vi "ma_MultitoneParamsCheck.vi"(4 "coerce frequencies?":bool, 5 "Relative error":dbl=1e-09 format="%0.3e", 6 "Phases":dbl[](array[numeric]) format="%0.2f", 7 "Samples":i32, 8 "error in (no error)":errorcluster, 9 "Sampling Rate":dbl format="%0.2f", 10 "Tone Frequencies":dbl[](array[numeric]) format="%0.2f", 11 "Tone Amplitudes":dbl[](array[numeric]) format="%0.2f") -> (0 "error out":errorcluster, 1 "Phases out":dbl[](array[numeric]) format="%0.2f", 2 "Tone Frequencies out":dbl[](array[numeric]) format="%0.2f", 3 "Tone Amplitudes out":dbl[](array[numeric]) format="%0.2f")   [LabVIEW 2020, in "NI_MAPro.lvlib"]
uses:
  NI_MAPro.lvlib
  NI_MABase.lvlib
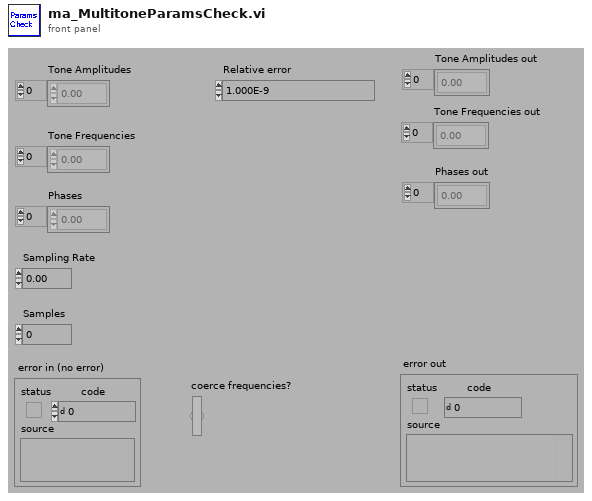
[diagram p1: front panel]
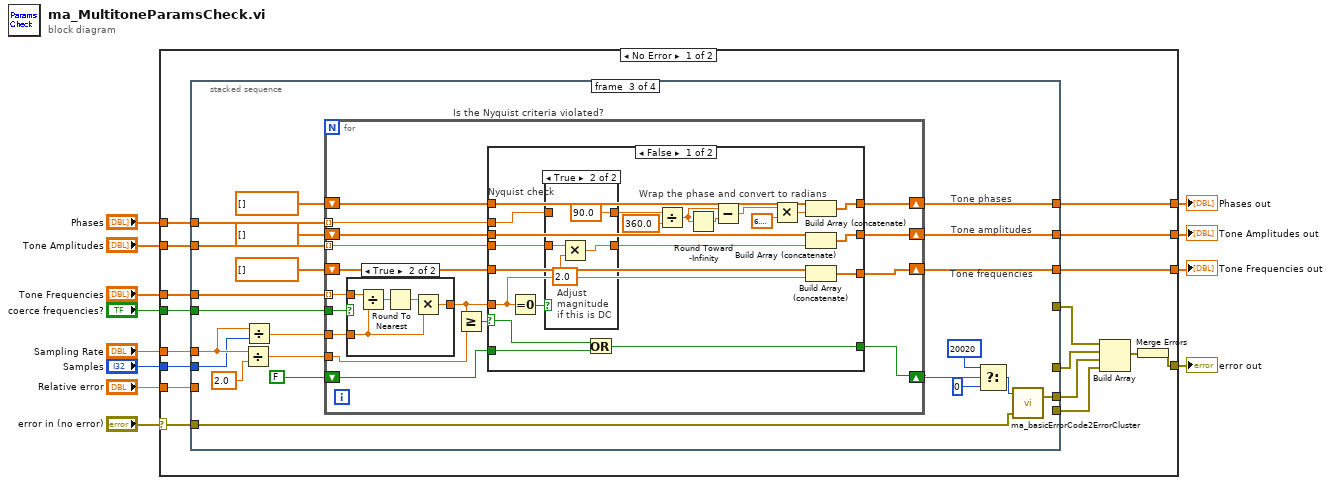
[diagram p0: block diagram]
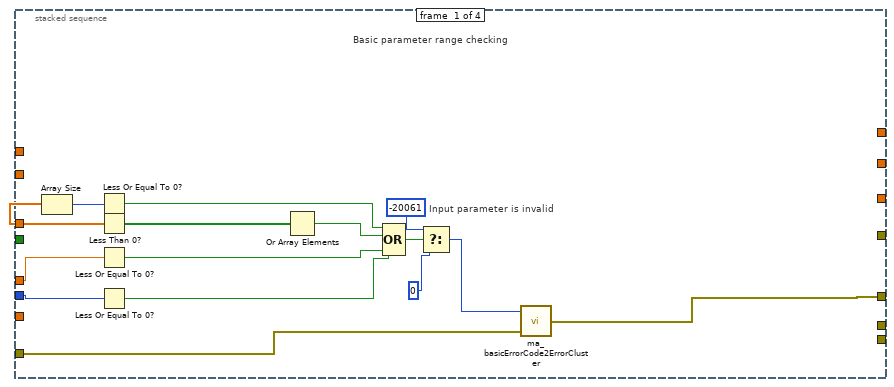
[diagram p2: hidden frame]
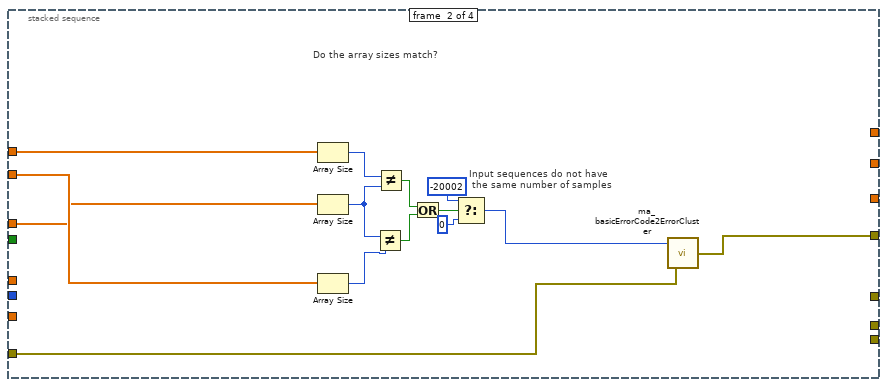
[diagram p3: hidden frame]
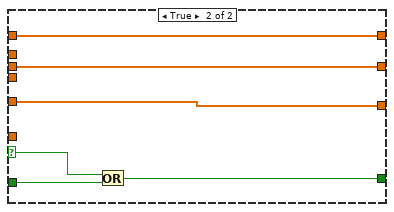
[diagram p6: hidden frame]
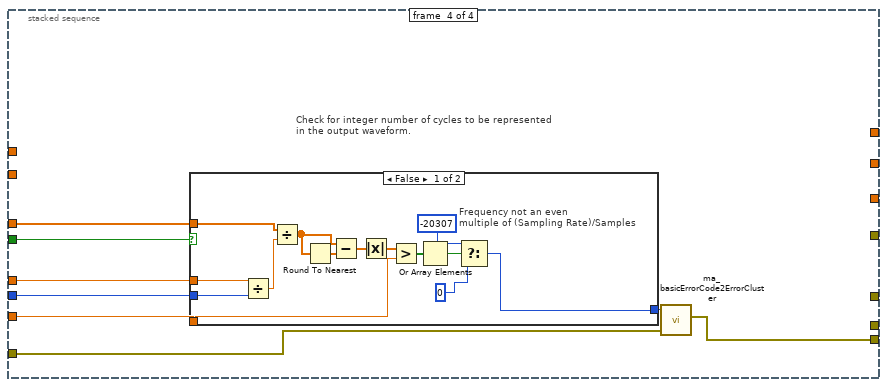
[diagram p7: hidden frame]
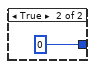
[diagram p8: hidden frame]
diagram:
  n1 = case shown="No Error" "error in (no error)" {
    selector: "error in (no error)" -> [w21 w159]
    tunnel: "Tone Frequencies" -> [w29 w160]
    tunnel: "Tone Amplitudes" -> [w28 w161]
    tunnel: "Sampling Rate" -> [w27 _]
    tunnel: "Samples" -> [w26 _]
    tunnel: "Phases" -> [w25 w162]
    tunnel: [w24 w162] -> w3
    tunnel: [w23 w161] -> w7
    tunnel: [w22 w160] -> w6
    tunnel: [w15 w159] -> w4
    tunnel: "Relative error" -> [w14 _]
    tunnel: "coerce frequencies?" -> [w13 _]
    frame No Error {
      n2 = stacked-sequence {
        tunnel: w29 -> [w34 w56 w80 w140]
        tunnel: w28 -> [_ w58 w79 _]
        tunnel: w27 -> [w43 _ w62 w143]
        tunnel: w26 -> [w44 _ w61 w142]
        tunnel: w14 -> [_ _ _ w141]
        tunnel: w25 -> [_ w57 w78 _]
        tunnel: [_ _ w67 _] -> w24
        tunnel: [_ _ w68 _] -> w23
        tunnel: [_ _ w71 _] -> w22
        tunnel: [w36 _ _ _] -> w19
        tunnel: w21 -> [w35 w50 w73 w139]
        tunnel: [_ w49 _ _] -> w20
        tunnel: [_ _ w72 _] -> w18
        tunnel: [_ _ _ w138] -> w17
        tunnel: w13 -> [_ _ w59 w136]
        frame #0 {
          # "Input parameter is invalid"
          # "Basic parameter range checking"
          n3 = Array Size(array=w34) -> (size(s)=w38:i32)
          n4 = Less Or Equal To 0?(x=w38) -> (x <= 0?=w37:bool)
          n5 = Less Than 0?(x=w34) -> (x < 0?=w42:bool[])
          n6 = Less Or Equal To 0?(x=w43) -> (x <= 0?=w41:bool)
          n7 = Less Or Equal To 0?(x=w44) -> (x <= 0?=w40:bool)
          n8 = Or Array Elements(Boolean array=w42) -> (logical OR=w39:bool)
          n9 = Compound Arithmetic op=OR(w37, w39, w41, w40) -> (w33:bool)
          n10 = Select(t=-20061 ("Bundle Element"), s=w33, f=0) -> (s? t:f=w30:i32)
          n11 = call "ma_basicErrorCode2ErrorCluster.vi"("error in (no error)"=w35, "Error Code"=w30) -> ("error out"=w36:errorcluster)  [unwired: 1 in]
        }
        frame #1 {
          # "Input sequences do not have\n the same number of samples"
          # "Do the array sizes match?"
          n12 = Array Size(array=w57) -> (size(s)=w52:i32)
          n13 = Array Size(array=w56) -> (size(s)=w53:i32)
          n14 = Array Size(array=w58) -> (size(s)=w51:i32)
          n15 = Not Equal?(x=w53, y=w51) -> (x != y?=w55:bool)
          n16 = Not Equal?(x=w52, y=w53) -> (x != y?=w54:bool)
          n17 = Or(x=w54, y=w55) -> (x .or. y?=w48:bool)
          n18 = Select(t=-20002 ("Bundle Element"), s=w48, f=0) -> (s? t:f=w45:i32)
          n19 = call "ma_basicErrorCode2ErrorCluster.vi"("error in (no error)"=w50, "Error Code"=w45) -> ("error out"=w49:errorcluster)  [unwired: 1 in]
        }
        frame #2 {
          # "Tone phases"
          # "Tone amplitudes"
          # "Tone frequencies"
          # "Is the Nyquist criteria violated?"
          # "Nyquist check"
          n20 = Divide(x=w62, y=2.0) -> (x/y=w69:dbl)
          n21 = Divide(x=w62, y=w61) -> (x/y=w60:dbl)
          n22 = for {
            tunnel: w69 -> [w85]
            tunnel: w80 -> [w84] mode=indexing
            shift-right: [w92] -> w71
            shift-left: dbl[] [] -> [w93]
            shift-right: [w94] -> w66
            shift-left: FALSE -> [w95]
            shift-right: [w89] -> w67
            shift-left: dbl[] [] -> [w90]
            shift-right: [w88] -> w68
            shift-left: dbl[] [] -> [w91]
            tunnel: w79 -> [w87] mode=indexing
            tunnel: w78 -> [w86] mode=indexing
            tunnel: w60 -> [w83]
            tunnel: w59 -> [w82]
            n23 = case shown="True" w82 {
              tunnel: w84 -> [w97 w102]
              tunnel: w83 -> [_ w99]
              tunnel: [w97 w98] -> w81
              frame False {
              }
              frame True {
                n24 = Divide(x=w102, y=w99) -> (x/y=w101:dbl)
                n25 = Round To Nearest(number=w101) -> (nearest integer value=w100:dbl)
                n26 = Multiply(x=w100, y=w99) -> (x*y=w98:dbl)
              }
            }
            n27 = Greater Or Equal?(x=w81, y=w85) -> (x >= y?=w96:bool)
            n28 = case shown="False" w96 {
              selector: w96 -> [w103 w130]
              tunnel: w95 -> [w117 w135]
              tunnel: [w116 w134] -> w94
              tunnel: w93 -> [w123 w133]
              tunnel: w81 -> [w115 _]
              tunnel: [w122 w133] -> w92
              tunnel: w91 -> [w120 w131]
              tunnel: w90 -> [w121 w132]
              tunnel: [w118 w132] -> w89
              tunnel: [w119 w131] -> w88
              tunnel: w87 -> [w113 _]
              tunnel: w86 -> [w112 _]
              frame False {
                # "Wrap the phase and convert to radians"
                n29 = Equal To 0?(x=w115) -> (x = 0?=w114:bool)
                n30 = case shown="True" w114 {
                  tunnel: w113 -> [w124 w129]
                  tunnel: w112 -> [w125 _]
                  tunnel: [w125 90.0 ("Phase")] -> w107
                  tunnel: [w124 w127] -> w108
                  frame False {
                  }
                  frame True {
                    # "Adjust \nmagnitude\nif this is DC"
                    n31 = Multiply(x=w129, y=2.0) -> (x*y=w127:dbl)
                  }
                }
                n32 = Or(x=w103, y=w117) -> (x .or. y?=w116:bool)
                n33 = Divide(x=w107, y=360.0) -> (x/y=w109:dbl)
                n34 = Round Toward -Infinity(1:w109) -> (0:w110:dbl)
                n35 = Subtract(x=w109, y=w110) -> (x-y=w105:dbl)
                n36 = Multiply(x=w105, y=6.283185307179586) -> (x*y=w106:dbl)
                n37 = Build Array (concatenate)(w121, w106) -> (w118:dbl[])
                n38 = Build Array (concatenate)(w120, w108) -> (w119:dbl[])
                n39 = Build Array (concatenate)(w123, w115) -> (w122:dbl[])
              }
              frame True {
                n40 = Or(x=w130, y=w135) -> (x .or. y?=w134:bool)
              }
            }
          }
          n41 = Select(t=20020 ("Bundle Element"), s=w66, f=0) -> (s? t:f=w63:i32)
          n42 = call "ma_basicErrorCode2ErrorCluster.vi"("error in (no error)"=w73, "Error Code"=w63) -> ("error out"=w72:errorcluster)  [unwired: 1 in]
        }
        frame #3 {
          # "Check for integer number of cycles to be represented\nin the output waveform."
          n43 = case shown="False" w136 {
            tunnel: w143 -> [w157 _]
            tunnel: w142 -> [w156 _]
            tunnel: w141 -> [w155 _]
            tunnel: w140 -> [w154 _]
            tunnel: [w144 0 ("Bundle Element")] -> w137
            frame False {
              # "Frequency not an even \nmultiple of (Sampling Rate)/Samples"
              n44 = Divide(x=w157, y=w156) -> (x/y=w150:dbl)
              n45 = Divide(x=w154, y=w150) -> (x/y=w151:dbl[])
              n46 = Round To Nearest(number=w151) -> (nearest integer value=w152:dbl[])
              n47 = Subtract(x=w151, y=w152) -> (x-y=w153:dbl[])
              n48 = Absolute Value(x=w153) -> (abs(x)=w149:dbl[])
              n49 = Greater?(x=w149, y=w155) -> (0:w148:bool[])
              n50 = Or Array Elements(Boolean array=w148) -> (logical OR=w147:bool)
              n51 = Select(t=-20307 ("Bundle Element"), s=w147, f=0) -> (s? t:f=w144:i32)
            }
            frame True {
            }
          }
          n52 = call "ma_basicErrorCode2ErrorCluster.vi"("error in (no error)"=w139, "Error Code"=w137) -> ("error out"=w138:errorcluster)  [unwired: 1 in]
        }
      }
      n53 = Build Array(w20, w19, w18, w17) -> (w16:errorcluster[])
      n54 = Merge Errors(w16) -> (w15:errorcluster)
    }
    frame Error {
    }
  }
  "error out" <- w4
  "Phases out" <- w3
  "Tone Amplitudes out" <- w7
  "Tone Frequencies out" <- w6
